vi "XYZ stage communication_coMD.vi"() -> ()   [LabVIEW 2012]
doc: "SciScan 1.2 160622"
uses:
  <vilib>/Utility/VariantDataType/Type.ctl
  CommonResource VIs/Timing/Timer Commands.ctl
  GFG/GFGstringGet.vi
  GFG/GFGnumericGet.vi
  GFG/GFGbooleanGet.vi
  GFG/GFG library.lvlib
  <vilib>/Utility/VariantDataType/VariantType.lvlib
panel:
  in  "stop":bool
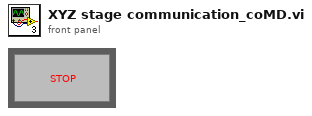
[diagram p1: front panel]
types:
  T1 = typedef "Timer Commands.ctl" = enum16{"Clear All", "Start", "Pause", "Check Time"}
  T2 = cluster{"moveXabs":dbl, "moveYabs":dbl, "moveZabs":dbl}
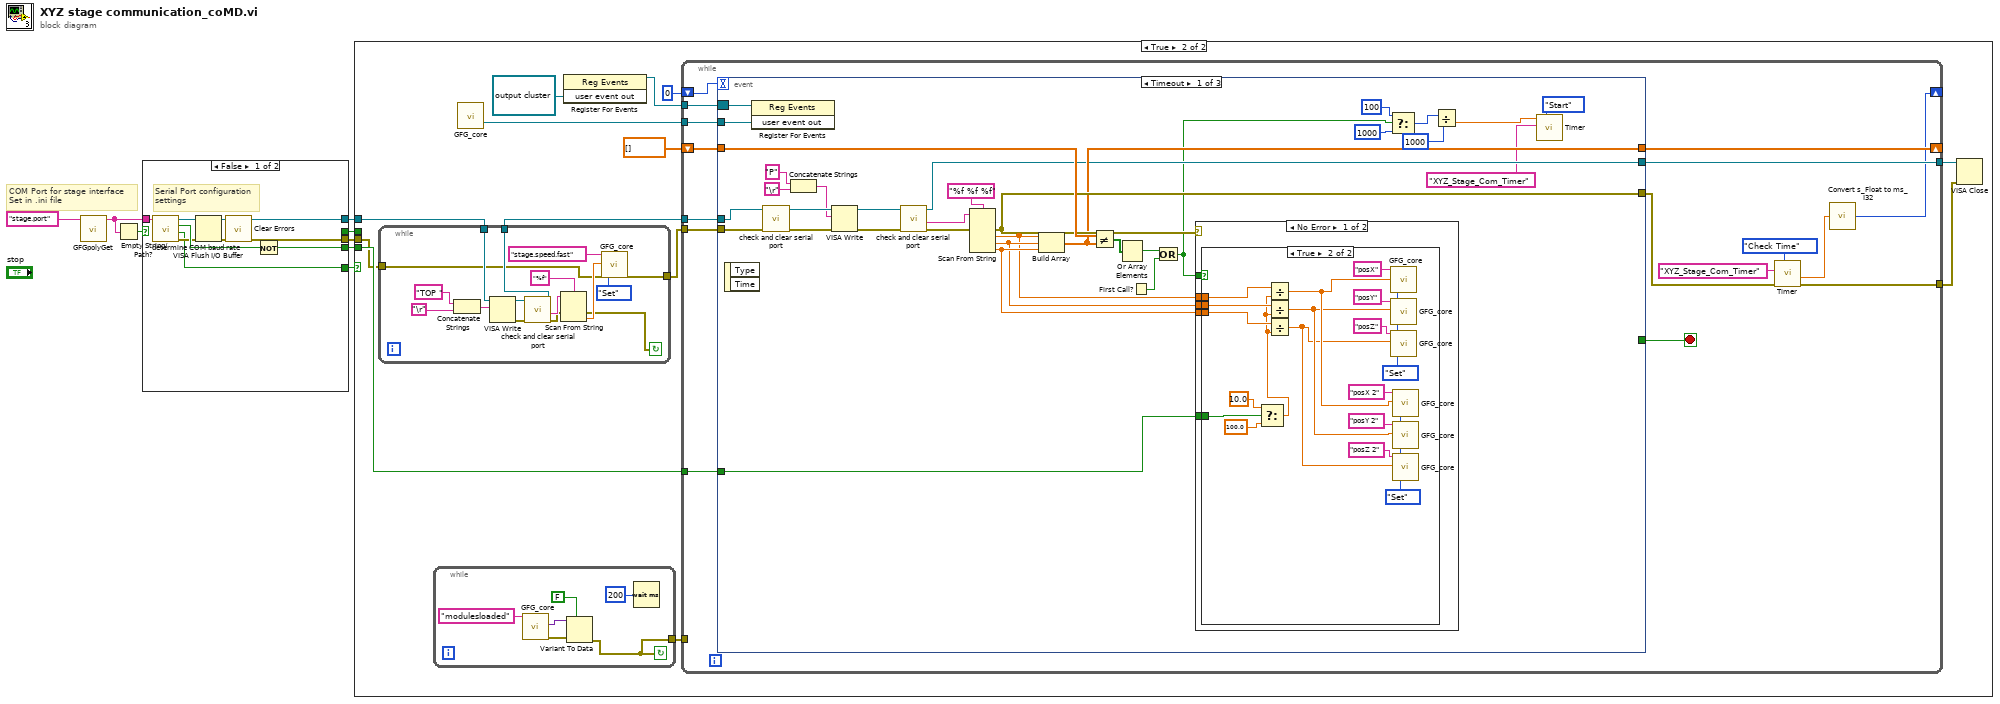
[diagram p0: block diagram]
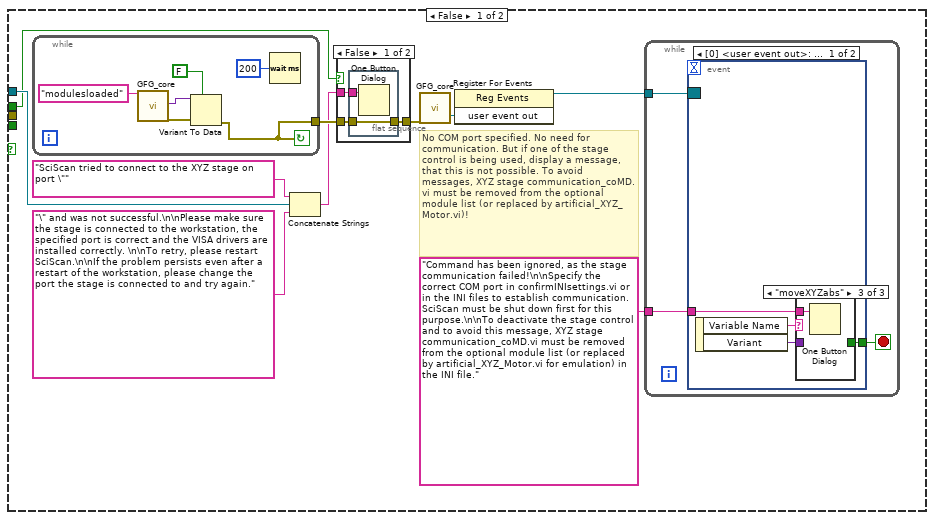
[diagram p3: hidden frame]
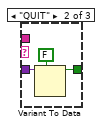
[diagram p6: hidden frame]
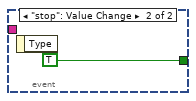
[diagram p7: hidden frame]
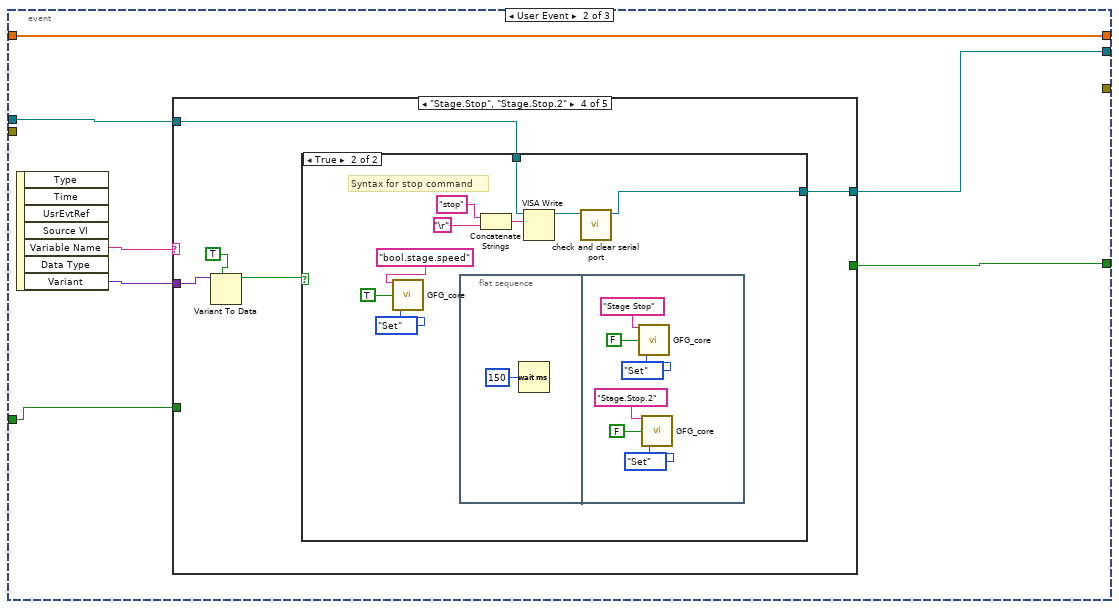
[diagram p10: hidden frame]
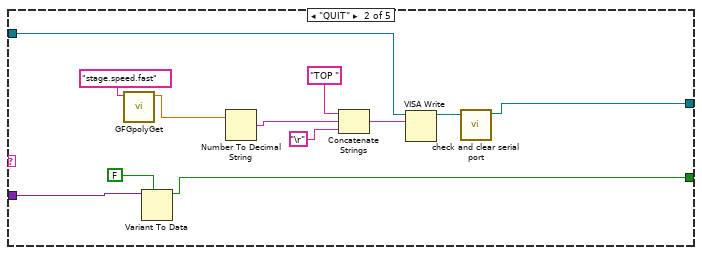
[diagram p12: hidden frame]
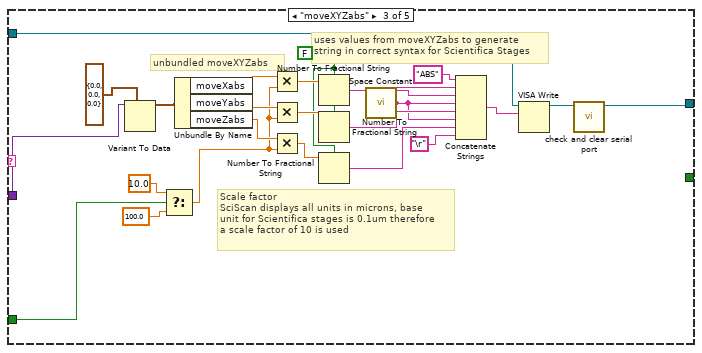
[diagram p13: hidden frame]
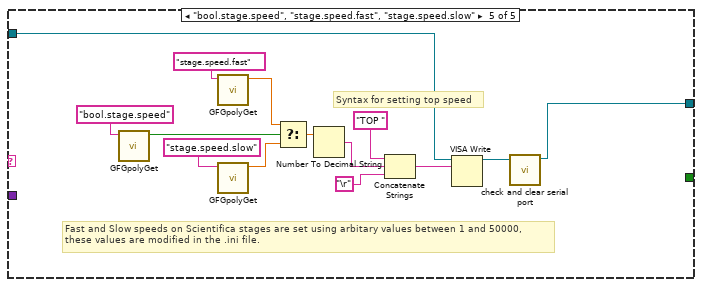
[diagram p15: hidden frame]
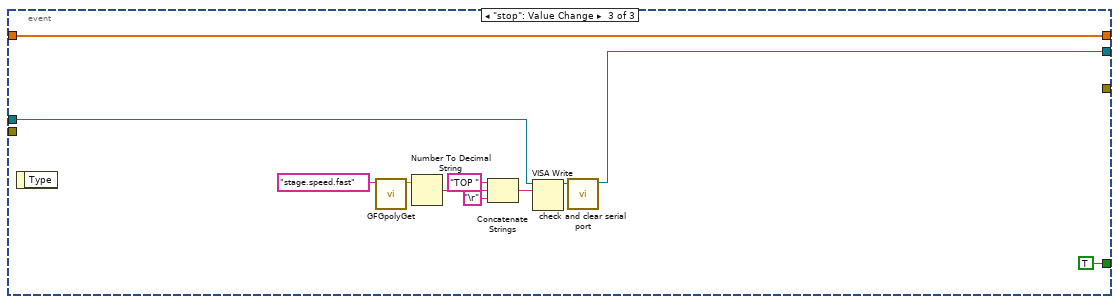
[diagram p16: hidden frame]
diagram:
  # "COM Port for stage interface\nSet in .ini file"
  n1 = call-poly "GFGpolyGet.vi"("Variable Name in"="stage.port") -> ("String"=w6:string)  [unwired: 9 in, 1 out]
  n2 = Empty String/Path?(string/path=w6) -> (empty?=w3:bool)
  n3 = case shown="False" w3 {
    selector: w3 -> [_ w18]
    tunnel: [w14 _] -> w7
    tunnel: w6 -> [w13 _]
    tunnel: [w12 _] -> w5
    tunnel: [w9 _] -> w4
    tunnel: [w11 _] -> w2
    tunnel: [_ w18] -> w1
    frame False {
      # "Serial Port configuration settings"
      n4 = call "determine COM baud rate.vi"("VISA resource name"=w13) -> ("error out"=w16:errorcluster, "Stage found?"=w11:bool, "card type (F for old cards, T for new cards)"=w17:bool, "VISA resource name out"=w15:refnum<visa-resource-name>)  [unwired: 7 in]
      n5 = VISA Flush I/O Buffer(VISA resource name=w15, error in (no error)=w16) -> (VISA resource name out=w12:refnum<visa-resource-name>, error out=w10:errorcluster)  [unwired: 1 in]
      n6 = call <vilib>:"Clear Errors.vi"("error in (no error)"=w10) -> ("error out"=w9:errorcluster)  [unwired: 6 in]
      n7 = Not(x=w17) -> (.not. x?=w14:bool)
    }
    frame True {
      # "No COM port specified. No need for communication. But if one of the stage control is being used, display a message, that this is not possible. To avoid messages, XYZ stage communication_coMD.vi must be removed from the optional module list (or replaced by artificial_XYZ_Motor.vi)!"
    }
  }
  n8 = case shown="True" w2 {
    tunnel: w7 -> [_ w55]
    tunnel: w5 -> [w21 w54]
    tunnel: w4 -> [_ w53]
    tunnel: w1 -> [w19 _]
    frame False {
      # "No COM port specified. No need for communication. But if one of the stage control is being used, display a message, that this is not possible. To avoid messages, XYZ stage communication_coMD.vi must be removed from the optional module list (or replaced by artificial_XYZ_Motor.vi)!"
      n9 = while {
        tunnel: [w35] -> w25
        stop <- w35 continue-if-true
        n10 = call "GFG_core.vi"("Variable Name in"="modulesloaded") -> ("Variant Out"=w36:variant, "error out"=w38:errorcluster)  [unwired: 12 in, 5 out]
        n11 = Variant To Data(error in=w38, type=FALSE, Variant=w36) -> (error out=w35:errorcluster)  [unwired: 1 out]
        n12 = Wait (ms)(milliseconds to wait=u32 200) -> ()  [unwired: 1 out]
      }
      n13 = Concatenate Strings("SciScan tried to connect to the XYZ stage on port \"" ("message"), w21, "\" and was not successful.\n\nPlease make sure the stage is connected to the workstation, the specified port is correct and the VISA drivers are installed correctly. \n\nTo retry, please restart SciScan.\n\nIf the problem persists even after a restart of the workstation, please change the port the stage is connected to and try again." ("message")) -> (w23:string)
      n14 = case shown="False" w19 {
        tunnel: w25 -> [w31 w34]
        tunnel: [w30 w34] -> w24
        tunnel: w23 -> [w29 _]
        frame False {
          n15 = flat-sequence {
            tunnel: w31 -> [w33]
            tunnel: [w33] -> w30
            tunnel: w29 -> [w32]
            frame #0 {
              n16 = One Button Dialog(message=w32) -> ()  [unwired: 1 in, 1 out]
            }
          }
        }
        frame True {
          # "No\nCOM\nselected."
        }
      }
      n17 = call "GFG_core.vi"("error in (no error)"=w24) -> ("user event out"=w26:refnum<user-event>)  [unwired: 12 in, 6 out]
      n18 = register-events(w26) -> (reference out=w28:refnum<event-registration>)  [unwired: 2 in, 1 out]
      n19 = while {
        tunnel: w28 -> [w42]
        tunnel: "Command has been ignored, as the stage communication failed!\n\nSpecify the correct COM port in confirmINIsettings.vi or in the INI files to establish communication. SciScan must be shut down first for this purpose.\n\nTo deactivate the stage control and to avoid this message, XYZ stage communication_coMD.vi must be removed from the optional module list (or replaced by artificial_XYZ_Motor.vi for emulation) in the INI file." ("message") -> [w41]
        stop <- w43 stop-if-true
        n20 = event shown="[0] <user event out>: User Event" {
          selector: w42 -> [_ _]
          dyn-events: _ -> [_ _]
          timeout: _ -> [_ _]
          tunnel: [w46 TRUE ("NewVal")] -> w43
          tunnel: w41 -> [w44 _]
          event User Event {
            n21 = event-data() -> ("Variable Name"=w45:string, "Variant"=w47:variant)  [unwired: 1 in]
            n22 = case shown="\"moveXYZabs\"" w45 {
              tunnel: [_ w48 _] -> w46
              tunnel: w47 -> [_ w50 _]
              tunnel: w44 -> [_ _ w51]
              frame Default {
              }
              frame "QUIT" {
                n23 = Variant To Data(type=FALSE ("NewVal"), Variant=w50) -> (data=w48:bool)  [unwired: 1 in, 1 out]
              }
              frame "moveXYZabs" {
                n24 = One Button Dialog(message=w51) -> ()  [unwired: 1 in, 1 out]
              }
            }
          }
          event "stop": Value Change {
            n25 = event-data() -> ()  [unwired: 1 in, 1 out]
          }
        }
      }
    }
    frame True {
      n26 = while {
        tunnel: w54 -> [w83]
        tunnel: [w82] -> w60
        tunnel: w53 -> [w75]
        tunnel: [w74] -> w58
        stop <- w76 continue-if-true
        n27 = Concatenate Strings("TOP " ("write buffer"), "\r") -> (w86:string)
        n28 = VISA Write(VISA resource name=w83, write buffer=w86) -> (VISA resource name out=w85:refnum<visa-resource-name>, error out=w73:errorcluster)  [unwired: 1 in, 1 out]
        n29 = call "check and clear serial port.vi"("error in (no error)"=w73, "VISA resource name in"=w85) -> ("error out"=w72:errorcluster, "read buffer"=w78:string, "VISA resource name out"=w82:refnum<visa-resource-name>)  [unwired: 6 in, 1 out]
        n30 = Scan From String(format string="%f", input string=w78, error in=w72) -> (error out=w76:errorcluster, output 1=w77:dbl)  [unwired: 2 in, 2 out]
        n31 = call "GFG_core.vi"("Variable Name in"="stage.speed.fast", "Variant in"=w77, "error in (no error)"=w75, "Action"=enum16{"Init", "Set", "Get"}."Set") -> ("error out"=w74:errorcluster)  [unwired: 9 in, 6 out]
      }
      n32 = while {
        tunnel: [w66] -> w57
        stop <- w66 continue-if-true
        n33 = call "GFG_core.vi"("Variable Name in"="modulesloaded") -> ("Variant Out"=w67:variant, "error out"=w69:errorcluster)  [unwired: 12 in, 5 out]
        n34 = Variant To Data(error in=w69, type=FALSE, Variant=w67) -> (error out=w66:errorcluster)  [unwired: 1 out]
        n35 = Wait (ms)(milliseconds to wait=u32 200) -> ()  [unwired: 1 out]
      }
      n36 = call "GFG_core.vi"() -> ("user event out"=w59:refnum<user-event>)  [unwired: 13 in, 6 out]
      n37 = register-events(refnum<user-event> refnum ("user event out")) -> (reference out=w61:refnum<event-registration>)  [unwired: 2 in, 1 out]
      n38 = while {
        tunnel: [w103] -> w63
        tunnel: w60 -> [w102]
        shift-right: [w101] -> _
        shift-left: dbl[] [] -> [w99]
        shift-right: [w90] -> _
        shift-left: 0 -> [w98]
        tunnel: w59 -> [w97]
        tunnel: w61 -> [w96]
        tunnel: w58 -> [w95]
        tunnel: w57 -> [_]
        tunnel: w55 -> [w94]
        tunnel: [w88] -> w56
        stop <- w100 stop-if-true
        n39 = event shown="[0] Timeout" {
          selector: w96 -> [w114 _ _]
          dyn-events: _ -> [_ _ _]
          timeout: w98 -> [_ _ _]
          tunnel: [w122 w162 w241] -> w103
          tunnel: w102 -> [w131 w163 w242]
          tunnel: [w134 w161 w240] -> w101
          tunnel: [_ w164 TRUE ("NewVal")] -> w100
          tunnel: w99 -> [w136 w161 w240]
          tunnel: w95 -> [w129 _ _]
          tunnel: [w135 _ _] -> w89
          tunnel: w97 -> [w113 _ _]
          tunnel: w94 -> [w109 w160 _]
          event Timeout {
            n40 = event-data() -> ()  [unwired: 1 in, 2 out]
            n41 = register-events(reference=w114, w113) -> ()  [unwired: 1 in, 2 out]
            n42 = call "check and clear serial port.vi"("error in (no error)"=w129, "VISA resource name in"=w131) -> ("error out"=w128:errorcluster, "VISA resource name out"=w130:refnum<visa-resource-name>)  [unwired: 6 in, 2 out]
            n43 = Concatenate Strings("P" ("write buffer"), "\r") -> (w120:string)
            n44 = VISA Write(VISA resource name=w130, write buffer=w120, error in (no error)=w128) -> (VISA resource name out=w124:refnum<visa-resource-name>, error out=w125:errorcluster)  [unwired: 1 out]
            n45 = call "check and clear serial port.vi"("error in (no error)"=w125, "VISA resource name in"=w124) -> ("error out"=w123:errorcluster, "read buffer"=w121:string, "VISA resource name out"=w122:refnum<visa-resource-name>)  [unwired: 6 in, 1 out]
            n46 = Scan From String(format string="%f %f %f", input string=w121, error in=w123) -> (error out=w135:errorcluster, output 1=w110:dbl, output 2=w111:dbl, output 3=w112:dbl)  [unwired: 4 in, 2 out]
            n47 = Build Array(w110, w111, w112) -> (w134:dbl[])
            n48 = Not Equal?(x=w136, y=w134) -> (x != y?=w133:bool[])
            n49 = Or Array Elements(Boolean array=w133) -> (logical OR=w117:bool)
            n50 = First Call?() -> (First Call?: T/F=w116:bool)
            n51 = Or(x=w117, y=w116) -> (x .or. y?=w115:bool)
            n52 = case shown="No Error" w135 {
              tunnel: w110 -> [w139 _]
              tunnel: w111 -> [w140 _]
              tunnel: w112 -> [w141 _]
              tunnel: w115 -> [w138 _]
              tunnel: w109 -> [w137 _]
              frame No Error {
                n53 = case shown="True" w138 {
                  tunnel: w141 -> [_ w156]
                  tunnel: w140 -> [_ w155]
                  tunnel: w139 -> [_ w154]
                  tunnel: w137 -> [_ w142]
                  frame False {
                  }
                  frame True {
                    w152 = enum16{"Init", "Set", "Get"}."Set" ("Action")
                    w153 = enum16{"Init", "Set", "Get"}."Set" ("Action")
                    n54 = Select(t=10.0 ("y"), s=w142, f=100.0 ("y")) -> (s? t:f=w143:dbl)
                    n55 = Divide(x=w154, y=w143) -> (x/y=w148:dbl)
                    n56 = Divide(x=w155, y=w143) -> (x/y=w147:dbl)
                    n57 = Divide(x=w156, y=w143) -> (x/y=w146:dbl)
                    n58 = call "GFG_core.vi"("Variable Name in"="posX", "Variant in"=w148, "Action"=w153) -> ()  [unwired: 10 in, 7 out]
                    n59 = call "GFG_core.vi"("Variable Name in"="posY", "Variant in"=w147, "Action"=w153) -> ()  [unwired: 10 in, 7 out]
                    n60 = call "GFG_core.vi"("Variable Name in"="posZ", "Variant in"=w146, "Action"=w153) -> ()  [unwired: 10 in, 7 out]
                    n61 = call "GFG_core.vi"("Variable Name in"="posX 2", "Variant in"=w148, "Action"=w152) -> ()  [unwired: 10 in, 7 out]
                    n62 = call "GFG_core.vi"("Variable Name in"="posY 2", "Variant in"=w147, "Action"=w152) -> ()  [unwired: 10 in, 7 out]
                    n63 = call "GFG_core.vi"("Variable Name in"="posZ 2", "Variant in"=w146, "Action"=w152) -> ()  [unwired: 10 in, 7 out]
                  }
                }
              }
              frame Error {
              }
            }
            n64 = Select(t=100, s=w115, f=1000) -> (s? t:f=w106:i32)
            n65 = Divide(x=w106, y=1000 ("x")) -> (x/y=w105:dbl)
            n66 = call "Timer.vi"("Timer Command"=Timer_Commands."Start", "VI name (Optional)"="XYZ_Stage_Com_Timer", "Set Time IN (s)"=w105) -> ()  [unwired: 3 in, 6 out]
          }
          event User Event {
            n67 = event-data() -> ("Variable Name"=w166:string, "Variant"=w165:variant)  [unwired: 1 in, 5 out]
            n68 = case shown="\"Stage.Stop\", \"Stage.Stop.2\"" w166 {
              tunnel: [_ w177 _ _ _] -> w164
              tunnel: w165 -> [_ w179 w190 w206 _]
              tunnel: w163 -> [w167 w173 w198 w208 w227]
              tunnel: [w167 w172 w192 w207 w226] -> w162
              tunnel: w160 -> [_ _ w181 _ _]
              frame "False", Default {
              }
              frame "QUIT" {
                n69 = call-poly "GFGpolyGet.vi"("Variable Name in"="stage.speed.fast") -> ("Numeric"=w170:dbl)  [unwired: 8 in, 2 out]
                n70 = Variant To Data(type=FALSE ("NewVal"), Variant=w179) -> (data=w177:bool)  [unwired: 1 in, 1 out]
                n71 = Number To Decimal String(number=w170) -> (decimal integer string=w168:string)  [unwired: 1 in]
                n72 = Concatenate Strings("TOP " ("write buffer"), w168, "\r") -> (w175:string)
                n73 = VISA Write(VISA resource name=w173, write buffer=w175) -> (VISA resource name out=w176:refnum<visa-resource-name>)  [unwired: 1 in, 2 out]
                n74 = call "check and clear serial port.vi"("VISA resource name in"=w176) -> ("VISA resource name out"=w172:refnum<visa-resource-name>)  [unwired: 7 in, 3 out]
              }
              frame "moveXYZabs" {
                w180 = FALSE ("use system decimal point (T)")
                # "Scale factor \nSciScan displays all units in microns, base \nunit for Scientifica stages is 0.1um therefore \na scale factor of 10 is used"
                # "unbundled moveXYZabs"
                # "uses values from moveXYZabs to generate\nstring in correct syntax for Scientifica Stages"
                n75 = Variant To Data(type=T2 {"moveXabs"=0.0, "moveYabs"=0.0, "moveZabs"=0.0} ("output cluster"), Variant=w190) -> (data=w188:T2)  [unwired: 1 in, 1 out]
                n76 = Select(t=10.0 ("y"), s=w181, f=100.0 ("y")) -> (s? t:f=w182:dbl)
                n77 = Unbundle By Name(w188) -> ("moveXabs"=w185:dbl, "moveYabs"=w186:dbl, "moveZabs"=w187:dbl)
                n78 = Multiply(x=w185, y=w182) -> (x*y=w196:dbl)
                n79 = Multiply(x=w186, y=w182) -> (x*y=w195:dbl)
                n80 = Multiply(x=w187, y=w182) -> (x*y=w194:dbl)
                n81 = Number To Fractional String(use system decimal point (T)=w180, number=w196) -> (F-format string=w203:string)  [unwired: 2 in]
                n82 = Number To Fractional String(use system decimal point (T)=w180, number=w195) -> (F-format string=w202:string)  [unwired: 2 in]
                n83 = Number To Fractional String(use system decimal point (T)=w180, number=w194) -> (F-format string=w201:string)  [unwired: 2 in]
                n84 = call <vilib>:"Space Constant.vi"() -> ("String"=w200:string)
                n85 = Concatenate Strings("ABS" ("string"), w200, w203, w200, w202, w200, w201, "\r") -> (w191:string)
                n86 = VISA Write(VISA resource name=w198, write buffer=w191) -> (VISA resource name out=w193:refnum<visa-resource-name>)  [unwired: 1 in, 2 out]
                n87 = call "check and clear serial port.vi"("VISA resource name in"=w193) -> ("VISA resource name out"=w192:refnum<visa-resource-name>)  [unwired: 7 in, 3 out]
              }
              frame "Stage.Stop", "Stage.Stop.2" {
                n88 = Variant To Data(type=TRUE, Variant=w206) -> (data=w204:bool)  [unwired: 1 in, 1 out]
                n89 = case shown="True" w204 {
                  tunnel: w208 -> [w209 w214]
                  tunnel: [w209 w213] -> w207
                  frame False {
                  }
                  frame True {
                    # "Syntax for stop command"
                    n90 = call "GFG_core.vi"("Variable Name in"="bool.stage.speed", "Variant in"=TRUE ("Boolean"), "Action"=enum16{"Init", "Set", "Get"}."Set") -> ()  [unwired: 10 in, 7 out]
                    n91 = flat-sequence {
                      frame #0 {
                        n92 = Wait (ms)(milliseconds to wait=u32 150) -> ()  [unwired: 1 out]
                      }
                      frame #1 {
                        n93 = call "GFG_core.vi"("Variable Name in"="Stage Stop", "Variant in"=FALSE ("Boolean"), "Action"=enum16{"Init", "Set", "Get"}."Set") -> ()  [unwired: 10 in, 7 out]
                        n94 = call "GFG_core.vi"("Variable Name in"="Stage.Stop.2", "Variant in"=FALSE ("Boolean"), "Action"=enum16{"Init", "Set", "Get"}."Set") -> ()  [unwired: 10 in, 7 out]
                      }
                    }
                    n95 = Concatenate Strings("stop" ("write buffer"), "\r") -> (w218:string)
                    n96 = VISA Write(VISA resource name=w214, write buffer=w218) -> (VISA resource name out=w217:refnum<visa-resource-name>)  [unwired: 1 in, 2 out]
                    n97 = call "check and clear serial port.vi"("VISA resource name in"=w217) -> ("VISA resource name out"=w213:refnum<visa-resource-name>)  [unwired: 7 in, 3 out]
                  }
                }
              }
              frame "bool.stage.speed", "stage.speed.fast", "stage.speed.slow" {
                # "Syntax for setting top speed"
                # "Fast and Slow speeds on Scientifica stages are set using arbitary values between 1 and 50000, \nthese values are modified in the .ini file."
                n98 = call-poly "GFGpolyGet.vi"("Variable Name in"="bool.stage.speed") -> ("Boolean Value OUT"=w230:bool)  [unwired: 9 in, 1 out]
                n99 = call-poly "GFGpolyGet.vi"("Variable Name in"="stage.speed.fast") -> ("Numeric"=w232:dbl)  [unwired: 8 in, 2 out]
                n100 = call-poly "GFGpolyGet.vi"("Variable Name in"="stage.speed.slow") -> ("Numeric"=w231:dbl)  [unwired: 8 in, 2 out]
                n101 = Select(t=w232, s=w230, f=w231) -> (s? t:f=w229:dbl)
                n102 = Number To Decimal String(number=w229) -> (decimal integer string=w228:string)  [unwired: 1 in]
                n103 = Concatenate Strings("TOP " ("write buffer"), w228, "\r") -> (w238:string)
                n104 = VISA Write(VISA resource name=w227, write buffer=w238) -> (VISA resource name out=w239:refnum<visa-resource-name>)  [unwired: 1 in, 2 out]
                n105 = call "check and clear serial port.vi"("VISA resource name in"=w239) -> ("VISA resource name out"=w226:refnum<visa-resource-name>)  [unwired: 7 in, 3 out]
              }
            }
          }
          event "stop": Value Change {
            n106 = event-data() -> ()  [unwired: 1 in, 1 out]
            n107 = call-poly "GFGpolyGet.vi"("Variable Name in"="stage.speed.fast") -> ("Numeric"=w246:dbl)  [unwired: 8 in, 2 out]
            n108 = Number To Decimal String(number=w246) -> (decimal integer string=w244:string)  [unwired: 1 in]
            n109 = Concatenate Strings("TOP " ("write buffer"), w244, "\r") -> (w249:string)
            n110 = VISA Write(VISA resource name=w242, write buffer=w249) -> (VISA resource name out=w250:refnum<visa-resource-name>)  [unwired: 1 in, 2 out]
            n111 = call "check and clear serial port.vi"("VISA resource name in"=w250) -> ("VISA resource name out"=w241:refnum<visa-resource-name>)  [unwired: 7 in, 3 out]
          }
        }
        n112 = call "Timer.vi"("Timer Command"=Timer_Commands."Check Time", "Error In"=w89, "VI name (Optional)"="XYZ_Stage_Com_Timer") -> ("Error Out"=w88:errorcluster, "Remaining Time (s)"=w91:dbl)  [unwired: 3 in, 4 out]
        n113 = call "Convert s_Float to ms_I32.vi"("Seconds IN (Float)"=w91) -> ("milliseconds OUT (I32)"=w90:i32)
      }
      n114 = VISA Close(VISA resource name=w63, error in (no error)=w56) -> ()  [unwired: 1 out]
    }
  }
